vi "EngineUI.vi"() -> ()   [LabVIEW 2013, in "PL Framework Configuration Tool.lvlib" / "Engine Parent Editor Node.lvclass"]
doc: "This VI is a template of the minimun components for a node UI.\nIt shows how to use the queue and the user event."
uses:
  Engine Parent Editor Node.lvclass
  <vilib>/NI/CEF/CEF_TreeControl/Node/NodeRef.ctl
  <vilib>/NI/CEF/CEF_TreeControl/Node/NISE_CEF_Node.lvclass
  <vilib>/NI/AMC/Message Queue.ctl
  <vilib>/NI/AMC/Message.ctl
  <vilib>/NI/Tools/Keyed Array/KeyedArray.ctl
  <vilib>/NI/CEF/CEF_TreeControl/Node/UserEventRef.ctl
  <vilib>/NI/CEF/CEF_TreeControl/Controls/EventCluster.ctl
  TBM Configuration Node/Get display name.vi
  <vilib>/NI/AMC/Create Single Message.vi
  <vilib>/NI/AMC/Update Message Routing Info.vi
  TBM Configuration Node/set display name.vi
  <vilib>/NI/Tag Bus Module Framework/root configuration/read metadata property.vi
  <vilib>/NI/AMC/Send Message.vi
  <vilib>/NI/Tag Bus Module Framework/root configuration/set metadata property.vi
  <vilib>/NI/AMC/AMC.lvlib
  <vilib>/NI/Tools/Keyed Array/Tools_KeyedArray.lvlib
  <vilib>/NI/CEF/CEF_TreeControl/NISE_CEF_TreeControl.lvlib
panel:
  in  "Name":string
  in  "user event":T1
  in  "main queue":T2
  in  "node ref":T3
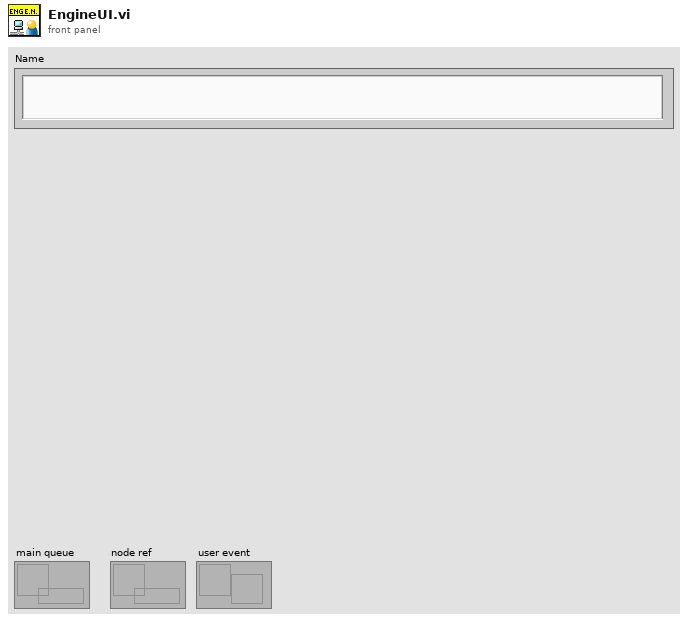
[diagram p1: front panel]
types:
  T1 = typedef "NISE_CEF_Node.lvclass/UserEventRef.ctl" = refnum<user-event>
  T2 = typedef "AMC.lvlib/Message Queue.ctl" = refnum<queue>
  T3 = typedef "NISE_CEF_Node.lvclass/NodeRef.ctl" = refnum<data-value>
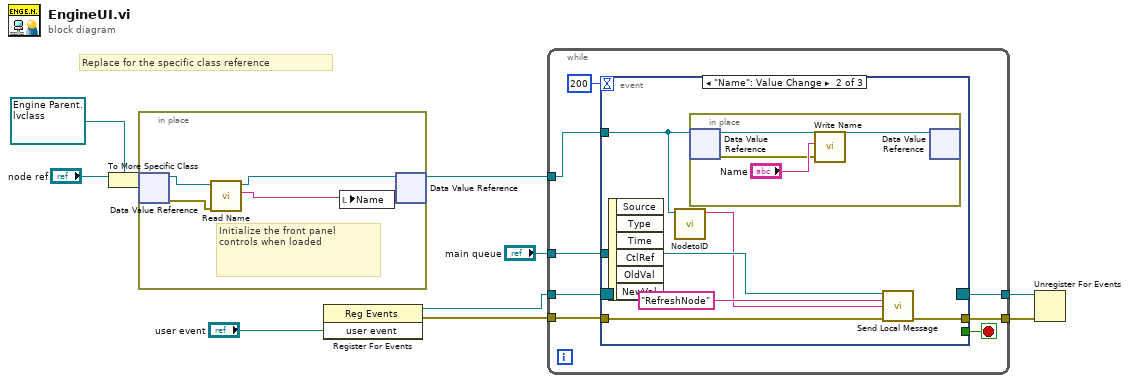
[diagram p0: block diagram]
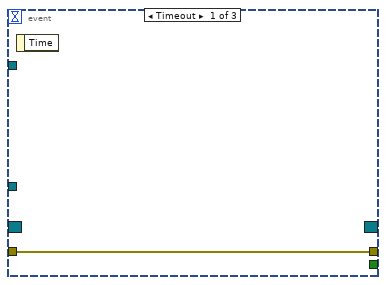
[diagram p2: hidden frame]
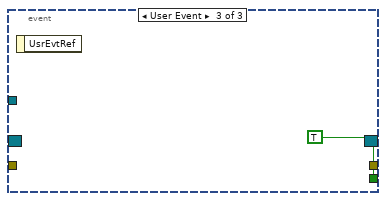
[diagram p3: hidden frame]
diagram:
  # "Replace for the specific class reference"
  n1 = To More Specific Class(target class=refnum<data-value> refnum ("data value reference"), reference="node ref") -> (specific class reference=w2:refnum<data-value>)  [unwired: 1 in, 1 out]
  n2 = in-place {
    # "Initialize the front panel  controls when loaded"
    n3 = in-place-dvr #1(w2) -> (w14:refnum<class "Engine Parent Editor Node.lvclass">, w13:errorcluster)
    n4 = call "Read Name.vi"("error in"=w13, "Engine in"=w14) -> ("Name"=w12:string, "Engine out"=w11:refnum<class "Engine Parent Editor Node.lvclass">)  [unwired: 7 in, 1 out]
    n5 = local write "Name"(w12) -> ()
    n6 = in-place-dvr #1(w11) -> (w10:refnum<data-value>)  [unwired: 1 out]
  }
  n7 = register-events("user event") -> (reference out=w7:refnum<event-registration>, error out=w4:errorcluster)  [unwired: 2 in]
  n8 = while {
    tunnel: w10 -> [w22]
    tunnel: "main queue" -> [w21]
    tunnel: w7 -> [w19]
    tunnel: [w18] -> w6
    tunnel: [w16] -> w5
    tunnel: w4 -> [w15]
    stop <- w17 stop-if-true
    n9 = event shown="[1] \"Name\": Value Change" {
      selector: w19 -> [_ _ _]
      dyn-events: [_ _ _] -> w18
      timeout: 200 -> [_ _ _]
      tunnel: w22 -> [_ w27 _]
      tunnel: w21 -> [_ w28 _]
      tunnel: [_ _ TRUE] -> w17
      tunnel: [w23 w25 _] -> w16
      tunnel: w15 -> [w23 w24 _]
      event Timeout {
        n10 = event-data() -> ()  [unwired: 1 in, 1 out]
      }
      event "Name": Value Change {
        n11 = event-data() -> ()  [unwired: 1 in, 6 out]
        n12 = call <vilib>:"NodetoID.vi"("node ref"=w27) -> ("ID"=w26:string)  [unwired: 9 in, 1 out]
        n13 = in-place {
          n14 = in-place-dvr #2(w27) -> (w33:refnum<class "Engine Parent Editor Node.lvclass">, w31:errorcluster)
          n15 = call "Write Name.vi"("error in"=w31, "Name"="Name", "Engine in"=w33) -> ("Engine out"=w30:refnum<class "Engine Parent Editor Node.lvclass">)  [unwired: 7 in, 1 out]
          n16 = in-place-dvr #2(w30) -> ()  [unwired: 2 out]
        }
        n17 = call <vilib>:"Send Local Message.vi"("message queue in"=w28, "message name"="RefreshNode" ("Message Name"), "message value"=w26, "error in"=w24) -> ("error out"=w25:errorcluster)  [unwired: 9 in, 2 out]
      }
      event User Event {
        n18 = event-data() -> ()  [unwired: 1 in, 1 out]
      }
    }
  }
  n19 = Unregister For Events(event registration refnum=w6, error in=w5) -> ()  [unwired: 1 out]
